vi "Config Relays.vi"(0 "VISA resource name":refnum<visa-resource-name>, 5 "Relay to \nConfigure (0: High)":u16(ring) items=["High", "Low"], 7 "Relay Mode (0: Off)":u16(ring) items=["Off", "Alarms", "Manual"], 9 "Manual Relay (F: Relay Off)":bool, 11 "error in (no error)":errorcluster) -> (4 "VISA resource name out":refnum<visa-resource-name>, 15 "error out":errorcluster)   [LabVIEW 2024, in "Lake Shore Cryotronics 340.lvlib"]
doc: "This VI configures the parameters of relay control."
uses:
  Lake Shore Cryotronics 340.lvlib
panel:
  # "Relay On\nRelay Off"
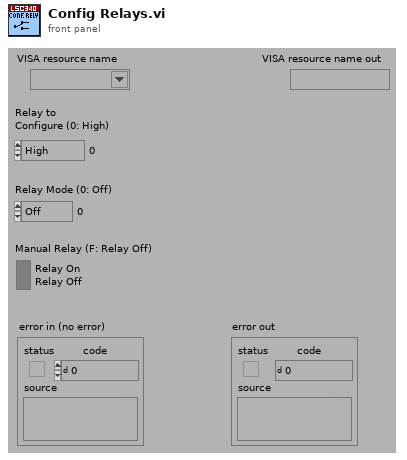
[diagram p1: front panel]
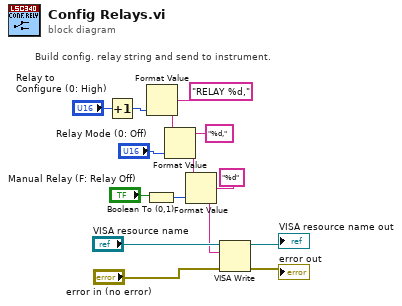
[diagram p0: block diagram]
diagram:
  # "Build config. relay string and send to instrument."
  n1 = Increment(x="Relay to \nConfigure (0: High)") -> (x+1=w9:u16)
  n2 = Boolean To (0,1)(Boolean="Manual Relay (F: Relay Off)") -> (0, 1=w12:i16)
  n3 = Format Value(format string="RELAY %d,", value (0)=w9) -> (output string=w7:string)  [unwired: 1 in]
  n4 = Format Value(string ("")=w7, format string="%d,", value (0)="Relay Mode (0: Off)") -> (output string=w8:string)
  n5 = Format Value(string ("")=w8, format string="%d", value (0)=w12) -> (output string=w1:string)
  n6 = VISA Write(VISA resource name="VISA resource name", write buffer=w1, error in (no error)="error in (no error)") -> (VISA resource name out=→"VISA resource name out":refnum<visa-resource-name>, error out=→"error out":errorcluster)  [unwired: 1 out]
